vi "TLB Native Dynamic Events ver 0.05e.vi"() -> ()   [LabVIEW 2018]
uses:
  Labview Training Phase 2/Enum Controls/States for Action Engine.ctl
  Type def/TLB event states.ctl
  Type def/TLB MHL States.ctl
  <vilib>/Studica/Studica Toolkit/Background/I2C Channel.ctl
  <vilib>/Studica/Studica Toolkit/NavX/NavX.lvlib
  <vilib>/myRIO/Common/Instrument Driver Framework/myRIO v1.0/AI/typedefs/AI Channels Enum.ctl
  <vilib>/myRIO/Common/Instrument Driver Framework/myRIO v1.0/AI/typedefs/AI Channels List.ctl
  <vilib>/Studica/Studica Toolkit/Background/Mxp Selection.ctl
  <vilib>/ptbypt/NI_PtbyPt.lvlib
  Type def/Type def.ctl
  Type def/Motor Control Cluster.ctl
panel:
  out "Object detected":bool
  out "Yaw":dbl
  in  "NavX Zero Yaw":bool
  out "NavX Info Out":T2
  out "LinearAcceleration":T3
  out "Displacement":T4
  out "YRPHfH":T5
  in  "y":dbl=-1.2 format="%#_13g"
  out "Distance":T6
  in  "Return to IDLE":bool
  out "Right IR Sensor":dbl
  out "Left IR Sensor":dbl
  out "CM":fxp<+,64,16>
  out "Ultrasonic sensor":dbl format="%0.2f"
  in  "xTargetSpeed":dbl
  in  "yTargetSpeed":dbl
  in  "wTargetSpeed":dbl
  out "Speed":T7
  in  "Reset Encoder 0":bool
  out "Action Queue Items":i32
  out "State Logic Queue Items":i32
  out "Action Queues items":string[](array[string])=["Hardware reset", "Software reset", ""]
  out "State logic":T8=enum."Task 2"
  out "Action State":string
  in  "Tasks Selector":string(combo)="Task 2"
  in  "Stop Queue":bool
  in  "Start Task":bool
  # "Test Programme written by Calvin Loke    Dated: 28 Aug 2019\nTest Programme revised by Dr Alex See   Dated 30 Aug 2019\n\nProgramme version:   TLB Native Dynamic Events ver 0.04b.vi"
  # "System Health Status Update"
  # "Sequence of Actions"
  # "Continuous (Repeated)"
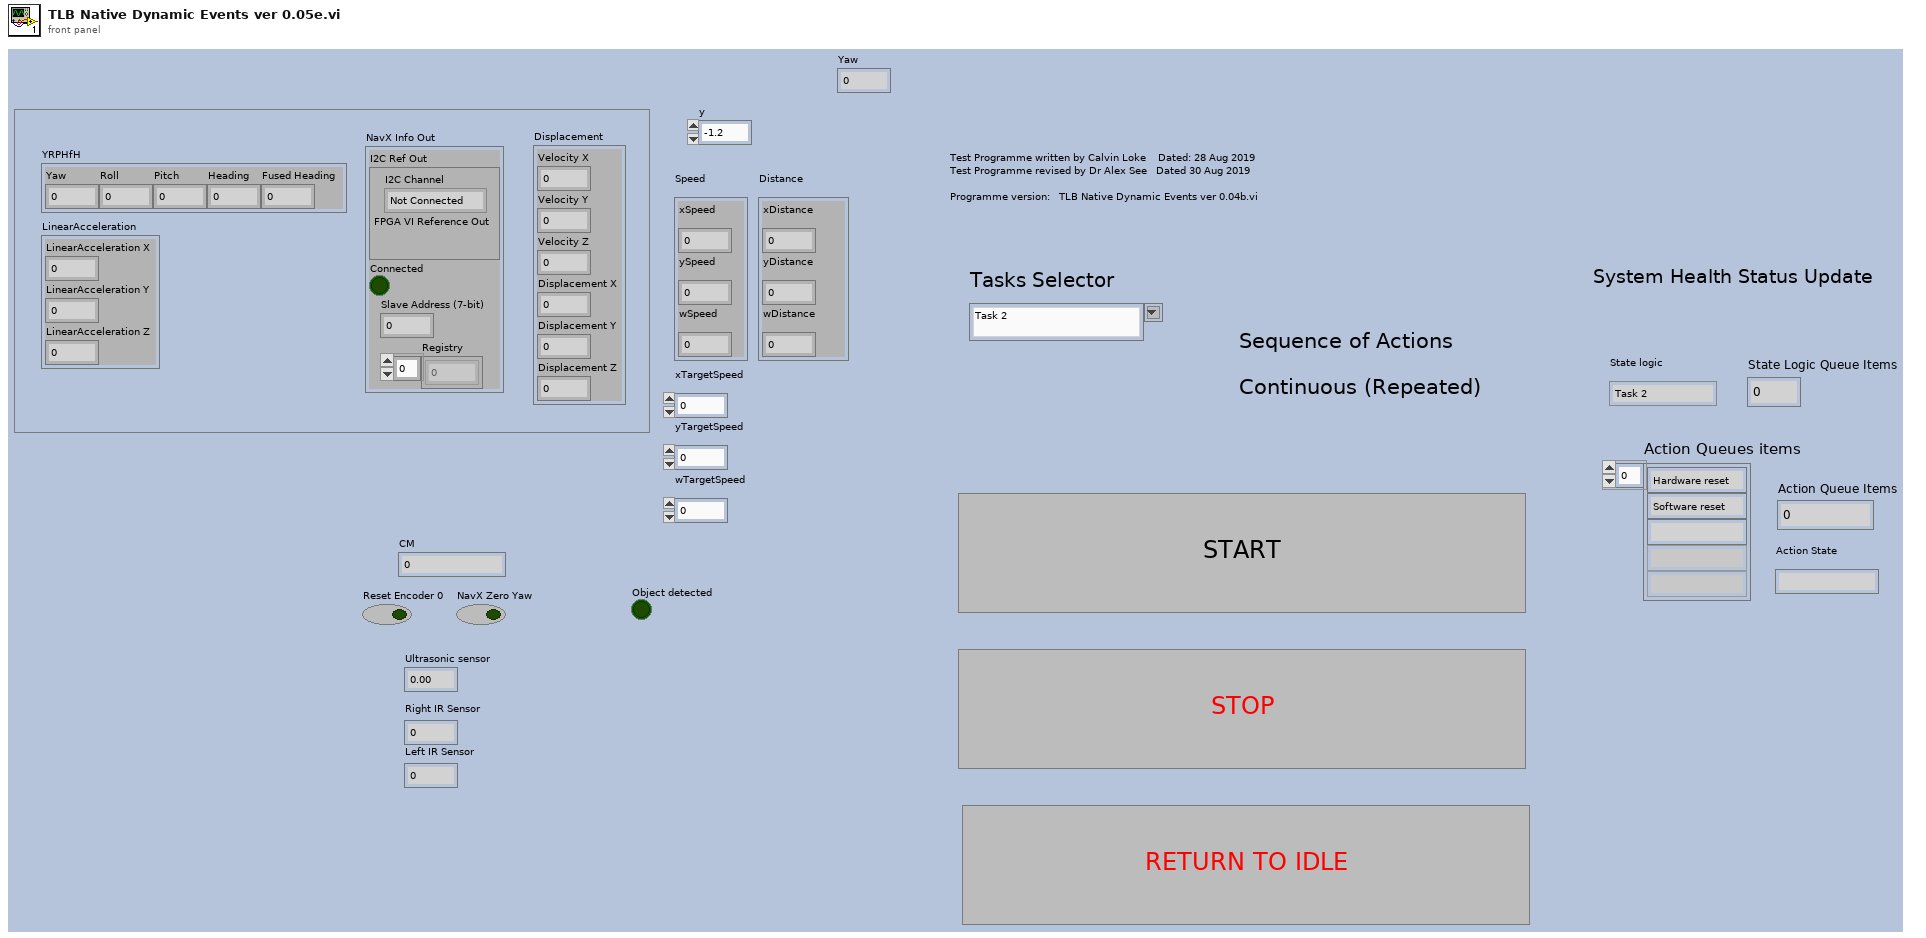
[diagram p1: front panel]
types:
  T1 = typedef "I2C Channel.ctl" = enum16{"Not Connected", "A", "B"}
  T2 = cluster{"I2C Ref Out":cluster{"I2C Channel":T1, "FPGA VI Reference Out":refnum<k20>}, "Connected":bool, "Slave Address (7-bit)":u8, "Registry":u8[]}
  T3 = cluster{"LinearAcceleration X":dbl, "LinearAcceleration Y":dbl, "LinearAcceleration Z":dbl}
  T4 = cluster{"Velocity X":dbl, "Velocity Y":dbl, "Velocity Z":dbl, "Displacement X":dbl, "Displacement Y":dbl, "Displacement Z":dbl}
  T5 = cluster{"Yaw":dbl, "Roll":dbl, "Pitch":dbl, "Heading":dbl, "Fused Heading":dbl}
  T6 = cluster{"xDistance":dbl, "yDistance":dbl, "wDistance":dbl}
  T7 = cluster{"xSpeed":dbl, "ySpeed":dbl, "wSpeed":dbl}
  T8 = typedef "TLB MHL States.ctl" = enum16{"None", "Startup", "Idle", "Processing", "Shutdown", "Reset", "Task 1", "Task 2", "Task 3", "Task 4", "Task 4a", "Task 4b", "Task 4c", "Task 4d", "Task 4e", "Task 4f", "Task 4g", "Task 4h", "Acquire image", "Wall follow mode", "Autodrive", "Autodrive a"}
  T9 = typedef "States for Action Engine.ctl" = enum16{"Initialize", "Write", "Read"}
  T10 = typedef "Motor Control Cluster.ctl" = cluster{"Vx":dbl, "Vy":dbl, "Vw":dbl}
  T11 = typedef "Type def.ctl" = cluster{"Front Ultrasonic Obstruct":bool, "Left Ultrasonic Obstruct":bool, "Right Ultrasonic Obstruct ":bool}
  T12 = typedef "TLB event states.ctl" = enum16{"Start Sequence", "Exit", "Start Task 1", "Start Task 2", "Start Task 3", "Start Task 4", "Camera vision", "Wall follow mode", "Idle", "Start Drive Straight"}
  T13 = typedef "Mxp Selection.ctl" = enum16{"MXP A", "MXP B"}
  T14 = typedef "AI Channels List.ctl" = T15[]
  T15 = typedef "AI Channels Enum.ctl" = enum16{"Not Connected", "AudioIn/Left", "AudioIn/Right", "C/AI0", "C/AI1", "A/AI0", "A/AI1", "A/AI2", "A/AI3", "A/AI4", "A/AI5", "A/AI6", "A/AI7", "B/AI0", "B/AI1", "B/AI2", "B/AI3", "B/AI4", "B/AI5", "B/AI6", "B/AI7", "AI/AI0", "AI/AI1", "AI/AI2", "AI/AI3", "A/AI0 (DIFF)", "A/AI1 (DIFF)", "A/AI2 (DIFF)", "A/AI3 (DIFF)", "B/AI0 (DIFF)", "B/AI1 (DIFF)", "B/AI2 (DIFF)", "B/AI3 (DIFF)"}
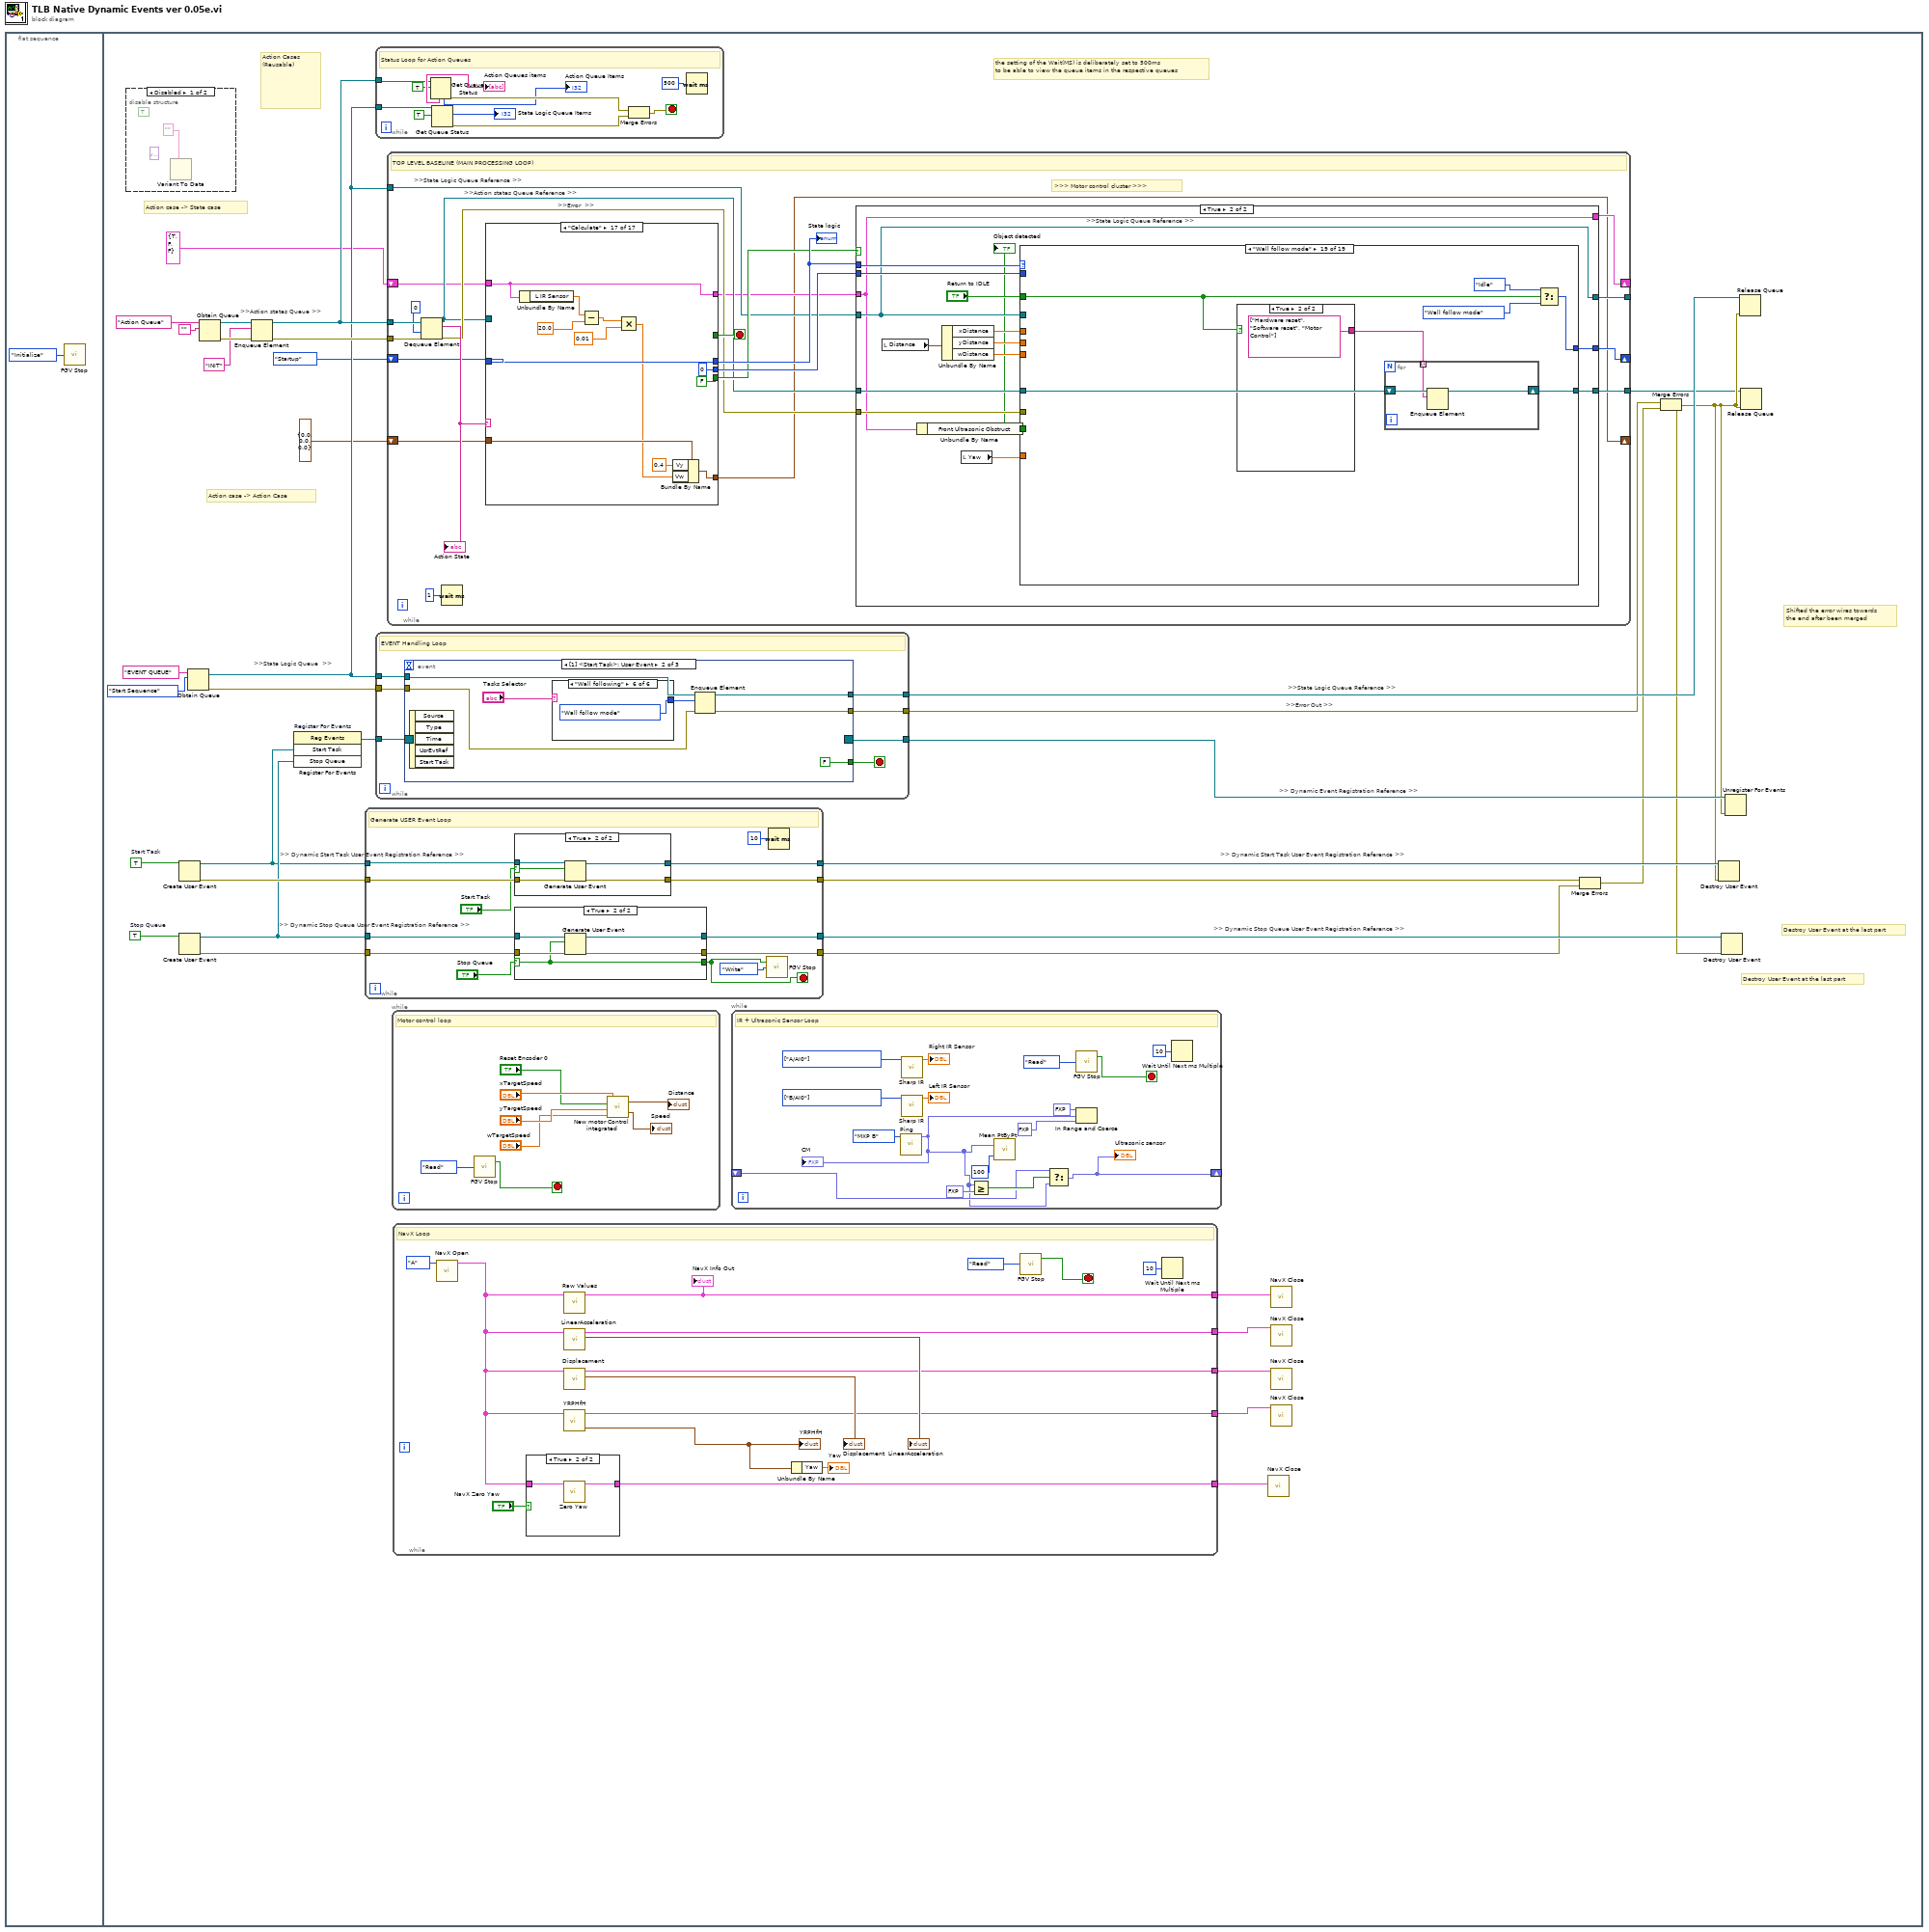
[diagram p0: block diagram]
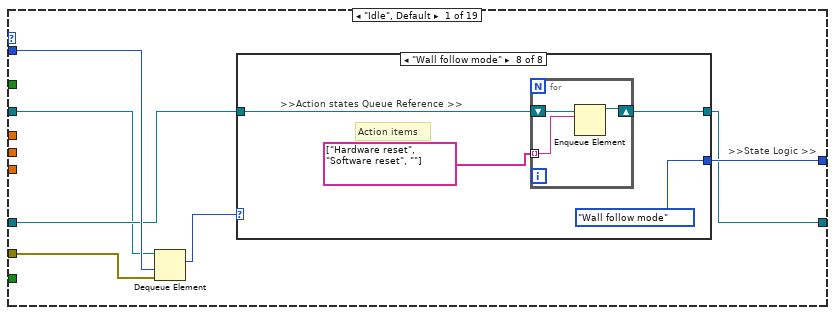
[diagram p5: hidden frame]
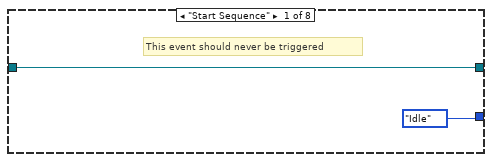
[diagram p6: hidden frame]
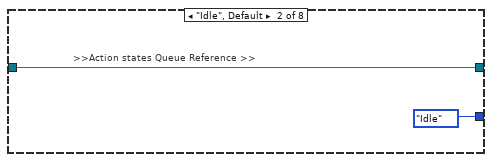
[diagram p7: hidden frame]
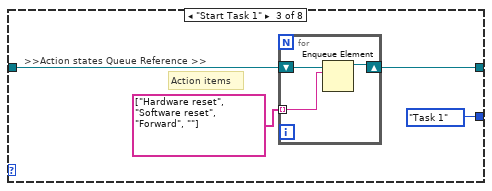
[diagram p8: hidden frame]
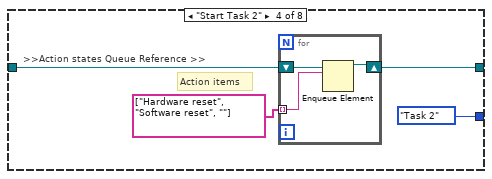
[diagram p9: hidden frame]
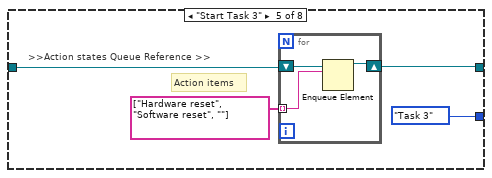
[diagram p10: hidden frame]
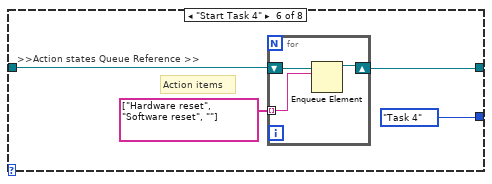
[diagram p11: hidden frame]
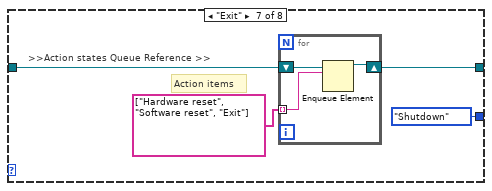
[diagram p12: hidden frame]
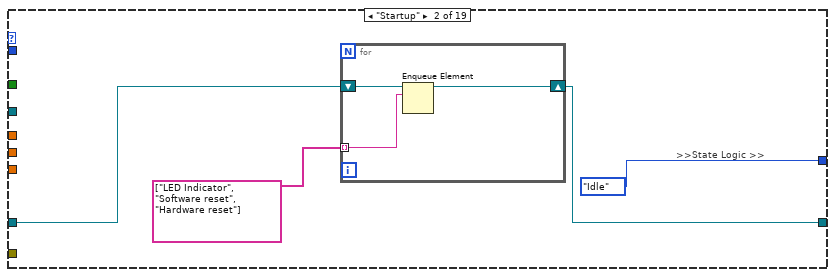
[diagram p13: hidden frame]
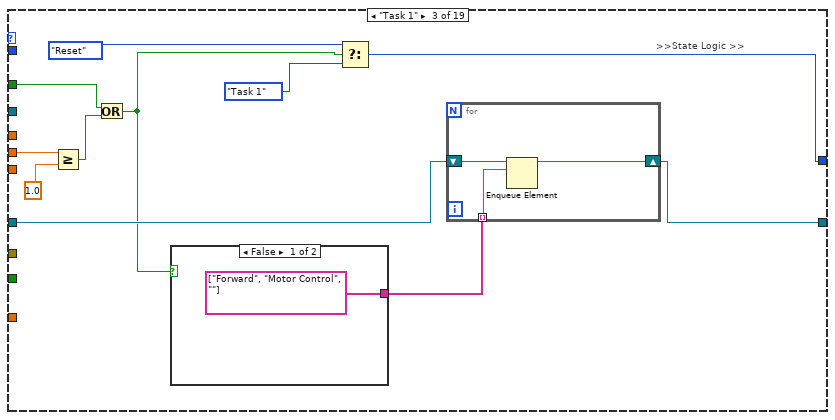
[diagram p14: hidden frame]
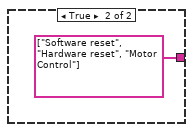
[diagram p15: hidden frame]
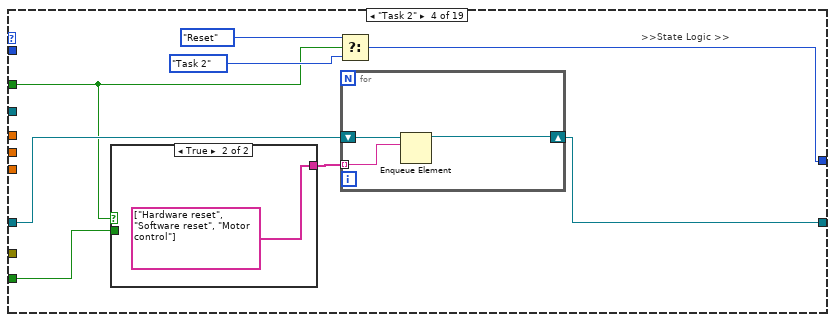
[diagram p16: hidden frame]
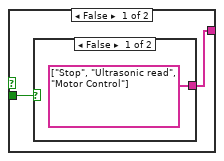
[diagram p17: hidden frame]
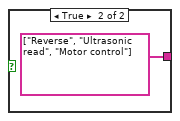
[diagram p18: hidden frame]
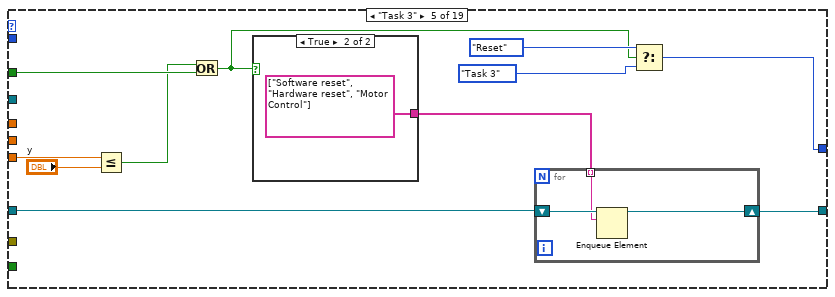
[diagram p19: hidden frame]
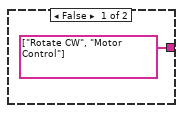
[diagram p20: hidden frame]
diagram:
  n1 = flat-sequence {
    frame #0 {
      n2 = call "FGV Stop.vi"("Init/Read/Write State"=States_for_Action_Engine."Initialize") -> ()  [unwired: 2 in, 2 out]
    }
    frame #1 {
      w37 = TRUE  # Stop Queue
      w36 = TRUE  # Start Task
      # "Action case -> Action Case"
      # "Action case -> State case"
      # "the setting of the Wait(MS) is deliberately set to 500ms\nto be able to view the queue items in the respective queues"
      # "Action Cases\n(Reusable)"
      # ">>Error Out >>"
      # ">> Dynamic Stop Queue User Event Registration Reference >>"
      # ">> Dynamic Start Task User Event Registration Reference >>"
      # ">> Dynamic Stop Queue User Event Registration Reference >>"
      # ">> Dynamic Start Task User Event Registration Reference >>"
      # ">> Dynamic Event Registration Reference >>"
      # ">>Action states Queue >>"
      # ">>State Logic Queue  >>"
      # ">>State Logic Queue Reference >>"
      # "Destroy User Event at the last part"
      # "Destroy User Event at the last part"
      # "Shifted the error wires towards\nthe end after been merged"
      n3 = disable-structure shown="Disabled" {
        frame Disabled {
          (unwired) variant
          (unwired) TRUE
          n4 = Variant To Data(type="") -> ()  [unwired: 2 in, 2 out]
        }
        frame Enabled {
        }
      }
      n5 = Create User Event(user event datatype=w36) -> (user event=w28:refnum<user-event>, error out=w33:errorcluster)  [unwired: 1 in]
      n6 = Create User Event(user event datatype=w37) -> (user event=w29:refnum<user-event>, error out=w32:errorcluster)  [unwired: 1 in]
      n7 = Obtain Queue(name (unnamed)="EVENT QUEUE", element data type=TLB_event_states."Start Sequence" ("Enum")) -> (queue out=w13:refnum<queue>, error out=w19:errorcluster)  [unwired: 3 in, 1 out]
      n8 = Obtain Queue(name (unnamed)="Action Queue", element data type="") -> (queue out=w22:refnum<queue>, error out=w18:errorcluster)  [unwired: 3 in, 1 out]
      n9 = Enqueue Element(queue=w22, element="INIT", error in (no error)=w18) -> (queue out=w14:refnum<queue>, error out=w17:errorcluster)  [unwired: 1 in, 1 out]
      n10 = register-events "Register For Events"(w28, w29) -> (reference out=w27:refnum<event-registration>)  [unwired: 2 in, 1 out]
      n11 = while {
        tunnel: w28 -> [w526]
        tunnel: w29 -> [w525]
        tunnel: [w524] -> w35
        tunnel: [w523] -> w34
        tunnel: w33 -> [w522]
        tunnel: [w521] -> w31
        tunnel: w32 -> [w520]
        tunnel: [w519] -> w30
        stop <- w515 stop-if-true
        # "Generate USER Event Loop"
        n12 = case shown="True" "Start Task" {
          selector: "Start Task" -> [_ w538]
          tunnel: w526 -> [w537 w542]
          tunnel: [w537 w541] -> w523
          tunnel: w522 -> [w536 w540]
          tunnel: [w536 w539] -> w521
          frame False {
          }
          frame True {
            n13 = Generate User Event(user event=w542, event data cluster=w538, error in=w540) -> (user event out=w541:refnum<user-event>, error out=w539:errorcluster)  [unwired: 1 in]
          }
        }
        n14 = case shown="True" "Stop Queue" {
          selector: "Stop Queue" -> [_ w531]
          tunnel: w525 -> [w530 w535]
          tunnel: [w530 w534] -> w524
          tunnel: w520 -> [w529 w533]
          tunnel: [w529 w532] -> w519
          tunnel: [FALSE w531] -> w515
          frame False {
          }
          frame True {
            n15 = Generate User Event(user event=w535, event data cluster=w531, error in=w533) -> (user event out=w534:refnum<user-event>, error out=w532:errorcluster)  [unwired: 1 in]
          }
        }
        n16 = call "FGV Stop.vi"("Init/Read/Write State"=States_for_Action_Engine."Write", "Input Node"=w515) -> ()  [unwired: 1 in, 2 out]
        n17 = Wait (ms)(milliseconds to wait=u32 10) -> ()  [unwired: 1 out]
      }
      n18 = while {
        tunnel: w14 -> [w89]
        tunnel: w13 -> [w86]
        stop <- w83 stop-if-true
        # "Status Loop for Action Queues"
        n19 = Get Queue Status(queue=w89, return elements? (F)=TRUE) -> (error out=w85:errorcluster, # elements in queue=→"Action Queue Items":i32, elements=→"Action Queues items":string[])  [unwired: 1 in, 5 out]
        n20 = Get Queue Status(queue=w86, return elements? (F)=TRUE) -> (# pending remove=→"State Logic Queue Items":i32, error out=w84:errorcluster)  [unwired: 1 in, 6 out]
        n21 = Merge Errors(w85, w84) -> (w83:errorcluster)
        n22 = Wait (ms)(milliseconds to wait=u32 500) -> ()  [unwired: 1 out]
      }
      n23 = while {
        tunnel: w27 -> [w489]
        tunnel: [w488] -> w26
        tunnel: w13 -> [w486]
        tunnel: [w485] -> w25
        tunnel: w19 -> [w484]
        tunnel: [w483] -> w16
        stop <- w487 stop-if-true
        # "EVENT Handling Loop"
        n24 = event shown="[1] <Start Task>: User Event" {
          selector: w489 -> [_ _ _]
          dyn-events: [_ _ _] -> w488
          timeout: _ -> [_ _ _]
          tunnel: [FALSE FALSE w514] -> w487
          tunnel: w486 -> [w494 w501 w512]
          tunnel: [w493 w500 w513] -> w485
          tunnel: w484 -> [w491 w497 w510]
          tunnel: [w490 w496 w509] -> w483
          event Timeout {
            n25 = event-data() -> ()  [unwired: 1 in, 3 out]
            n26 = Enqueue Element(queue=w494, element=TLB_event_states."Idle" ("Enum"), error in (no error)=w491) -> (queue out=w493:refnum<queue>, error out=w490:errorcluster)  [unwired: 1 in, 1 out]
          }
          event User Event {
            n27 = event-data() -> ()  [unwired: 1 in, 5 out]
            n28 = case shown="\"Wall following\"" "Tasks Selector" {
              tunnel: [TLB_event_states."Idle" ("Enum") TLB_event_states."Start Task 1" ("Enum") TLB_event_states."Start Task 2" ("Enum") TLB_event_states."Start Task 3" ("Enum") TLB_event_states."Start Task 4" ("Enum") TLB_event_states."Wall follow mode" ("Enum")] -> w498
              frame Default {
              }
              frame "Task 1" {
              }
              frame "Task 2" {
              }
              frame "Task 3" {
              }
              frame "Task 4" {
              }
              frame "Wall following" {
              }
            }
            n29 = Enqueue Element(queue=w501, element=w498, error in (no error)=w497) -> (queue out=w500:refnum<queue>, error out=w496:errorcluster)  [unwired: 1 in, 1 out]
          }
          event User Event {
            n30 = event-data() -> ("Stop Queue"=w514:bool)  [unwired: 1 in, 4 out]
            n31 = Enqueue Element At Opposite End(queue=w512, element=TLB_event_states."Exit" ("Enum"), error in (no error)=w510) -> (queue out=w513:refnum<queue>, error out=w509:errorcluster)  [unwired: 1 in, 1 out]
          }
        }
      }
      n32 = while {
        tunnel: w13 -> [w100]
        shift-right: [w105] -> _
        shift-left: TLB_MHL_States."Startup" ("Enum") -> [w97]
        tunnel: w14 -> [w110]
        tunnel: w17 -> [w108]
        tunnel: [w107] -> _
        tunnel: [w106] -> w11
        shift-right: [w94] -> _
        shift-left: T11 {"Front Ultrasonic Obstruct"=TRUE, "Left Ultrasonic Obstruct"=FALSE, "Right Ultrasonic Obstruct "=FALSE} -> [w96]
        shift-right: [w92] -> _
        shift-left: T10 {"Vx"=0.0, "Vy"=0.0, "Vw"=0.0} -> [w93]
        stop <- w103 stop-if-true
        # ">>> Motor control cluster >>>"
        # ">>Error  >>"
        # ">>Action states Queue Reference >>"
        # ">>State Logic Queue Reference >>"
        # "TOP LEVEL BASELINE (MAIN PROCESSING LOOP)"
        n33 = Dequeue Element(queue=w110, timeout in ms (-1)=0, error in (no error)=w108) -> (queue out=w98:refnum<queue>, element=w109:string, error out=w99:errorcluster)  [unwired: 1 out]
        "Action State" <- w109
        n34 = Wait (ms)(milliseconds to wait=u32 1) -> ()  [unwired: 1 out]
        n35 = case shown="\"Calculate\"" w109 {
          tunnel: [w349 w356 w361 w369 w378 w388 w397 w404 w415 w423 w431 w439 w448 TLB_MHL_States."Shutdown" ("Enum") w463 w467 w481] -> w111
          tunnel: [w348 0 0 0 0 0 0 0 0 0 0 0 0 0 0 0 0] -> w104
          tunnel: [_ _ _ _ _ _ _ _ _ _ _ _ _ TRUE _ _ _] -> w103
          tunnel: [TRUE FALSE FALSE FALSE FALSE FALSE FALSE FALSE FALSE FALSE FALSE FALSE FALSE FALSE FALSE FALSE FALSE] -> w102
          tunnel: w98 -> [_ _ _ _ _ _ _ _ _ _ _ _ _ _ _ _ _]
          tunnel: w97 -> [w349 w356 w361 w369 w378 w388 w397 w404 w415 w423 w431 w439 w448 _ w463 w467 w481]
          tunnel: w96 -> [w346 w353 w358 w365 w374 w383 w392 w401 w410 w419 w432 w436 w443 w450 w462 w470 w482]
          tunnel: [w346 w353 w358 w365 w374 w383 w392 w401 w410 w419 w432 w435 w443 w450 w459 w469 w482] -> w95
          tunnel: w93 -> [w345 w352 w357 w363 w372 w381 w391 w399 w409 w417 w425 w433 w442 w449 w455 w464 w473]
          tunnel: [w345 w352 w357 w364 w373 w382 w390 w400 w408 w418 w425 w433 w440 w449 w455 w464 w474] -> w92
          frame "No action", Default {
            n36 = case shown="\"Idle\"" w349 {
              tunnel: [0 100] -> w348
              frame "Startup", Default {
              }
              frame "Idle" {
              }
            }
          }
          frame "Init" {
            # ">>State Logic  >>"
          }
          frame "LED Indicator" {
          }
          frame "Forward" {
            n37 = local write "Reset Encoder 0"(FALSE ("Reset Encoder 0")) -> ()
            n38 = local write "NavX Zero Yaw"(FALSE ("NavX Zero Yaw")) -> ()
            n39 = Bundle By Name(cluster=w363, "Vy"=0.6) -> (w364:T10)
          }
          frame "Reverse" {
            n40 = local write "NavX Zero Yaw"(FALSE ("NavX Zero Yaw")) -> ()
            n41 = local write "Reset Encoder 0"(FALSE ("Reset Encoder 0")) -> ()
            n42 = Bundle By Name(cluster=w372, "Vy"=-0.6) -> (w373:T10)
          }
          frame "Right" {
            n43 = local write "NavX Zero Yaw"(FALSE ("NavX Zero Yaw")) -> ()
            n44 = local write "Reset Encoder 0"(FALSE ("Reset Encoder 0")) -> ()
            n45 = Bundle By Name(cluster=w381, "Vx"=0.6) -> (w382:T10)
          }
          frame "Left" {
            n46 = Bundle By Name(cluster=w391, "Vx"=-0.6) -> (w390:T10)
            n47 = local write "NavX Zero Yaw"(FALSE ("NavX Zero Yaw")) -> ()
            n48 = local write "Reset Encoder 0"(FALSE ("Reset Encoder 0")) -> ()
          }
          frame "Rotate CW" {
            n49 = local write "NavX Zero Yaw"(FALSE ("NavX Zero Yaw")) -> ()
            n50 = local write "Reset Encoder 0"(FALSE ("Reset Encoder 0")) -> ()
            n51 = Bundle By Name(cluster=w399, "Vw"=-0.3) -> (w400:T10)
          }
          frame "Rotate ACW" {
            n52 = local write "Reset Encoder 0"(FALSE ("Reset Encoder 0")) -> ()
            n53 = local write "NavX Zero Yaw"(FALSE ("NavX Zero Yaw")) -> ()
            n54 = Bundle By Name(cluster=w409, "Vw"=0.15) -> (w408:T10)
          }
          frame "Stop" {
            w416 = 0.0
            n55 = local write "NavX Zero Yaw"(FALSE ("NavX Zero Yaw")) -> ()
            n56 = local write "Reset Encoder 0"(FALSE ("Reset Encoder 0")) -> ()
            n57 = Bundle By Name(cluster=w417, "Vx"=w416, "Vy"=w416, "Vw"=w416) -> (w418:T10)
          }
          frame "Motor control" {
            # "Replace with FGV"
            n58 = Unbundle By Name(w425) -> ("Vx"=w428:dbl, "Vy"=w427:dbl, "Vw"=w426:dbl)
            n59 = local write "xTargetSpeed"(w428) -> ()
            n60 = local write "yTargetSpeed"(w427) -> ()
            n61 = local write "wTargetSpeed"(w426) -> ()
          }
          frame "Software reset" {
            w434 = FALSE ("NavX Zero Yaw")
            n62 = local write "NavX Zero Yaw"(w434) -> ()
            n63 = Bundle By Name(cluster=w436, "Front Ultrasonic Obstruct"=w434) -> (w435:T11)
          }
          frame "Hardware reset" {
            w441 = 0.0
            n64 = local write "Reset Encoder 0"(TRUE ("Reset Encoder 0")) -> ()
            n65 = local write "NavX Zero Yaw"(TRUE ("NavX Zero Yaw")) -> ()
            n66 = Bundle By Name(cluster=w442, "Vx"=w441, "Vy"=w441, "Vw"=w441) -> (w440:T10)
          }
          frame "Exit" {
          }
          frame "Ultrasonic read" {
            # "Object detection"
            n67 = local read "Ultrasonic sensor"() -> (w458:dbl)
            n68 = Less Or Equal?(x=w458, y=20.0) -> (x <= y?=w456:bool)
            n69 = Bundle By Name(cluster=w462, "Front Ultrasonic Obstruct"=w456) -> (w459:T11)
          }
          frame "IR Sensor Read" {
            n70 = local read "Left IR Sensor"() -> (w468:dbl)
            n71 = Bundle By Name(cluster=w470, "L IR Sensor"=w468) -> (w469:T11)
          }
          frame "Calculate" {
            n72 = Unbundle By Name(w482) -> ("L IR Sensor"=w478:dbl)
            n73 = Subtract(x=w478, y=20.0) -> (x-y=w476:dbl)
            n74 = Multiply(x=w476, y=0.01) -> (x*y=w472:dbl)
            n75 = Bundle By Name(cluster=w473, "Vy"=0.4, "Vw"=w472) -> (w474:T10)
          }
        }
        "State logic" <- w111
        n76 = case shown="True" w102 {
          tunnel: w111 -> [w115 w131]
          tunnel: w100 -> [w116 w125]
          tunnel: w98 -> [w114 w130]
          tunnel: [w116 w125] -> w107
          tunnel: [w114 w129] -> w106
          tunnel: [w115 w128] -> w105
          tunnel: w99 -> [_ w127]
          tunnel: w104 -> [_ w126]
          tunnel: w95 -> [w113 w117]
          tunnel: [w113 w117] -> w94
          frame False {
          }
          frame True {
            # ">>State Logic Queue Reference >>"
            n77 = local read "Distance"() -> (w123:T6)
            n78 = Unbundle By Name(w117) -> ("Front Ultrasonic Obstruct"=w118:bool)
            "Object detected" <- w118
            n79 = Unbundle By Name(w123) -> ("xDistance"=w120:dbl, "yDistance"=w122:dbl, "wDistance"=w121:dbl)
            n80 = local read "Yaw"() -> (w119:dbl)
            n81 = case shown="\"Wall follow mode\"" w131 {
              tunnel: w125 -> [w132 _ _ _ _ _ _ _ _ _ _ _ _ _ _ _ _ _ _]
              tunnel: w130 -> [w134 w186 w198 w211 w233 w242 w256 w271 w284 w297 w308 w314 w317 w323 w326 w328 w330 w332 w335]
              tunnel: [w133 w185 w197 w212 w232 w243 w255 w270 w283 w296 w307 w314 w316 w323 w326 w328 w330 w332 w336] -> w129
              tunnel: [w137 TLB_MHL_States."Idle" ("Enum") w200 w213 w229 w246 w258 w269 w285 w295 TLB_MHL_States."Idle" ("Enum") TLB_MHL_States."Reset" ("Enum") TLB_MHL_States."Shutdown" ("Enum") TLB_MHL_States."Reset" ("Enum") TLB_MHL_States."Idle" ("Enum") TLB_MHL_States."Idle" ("Enum") TLB_MHL_States."Idle" ("Enum") TLB_MHL_States."Idle" ("Enum") w338] -> w128
              tunnel: w127 -> [w135 _ _ _ _ _ _ _ _ _ _ _ _ _ _ _ _ _ _]
              tunnel: w126 -> [w136 _ _ _ _ _ _ _ _ _ _ _ _ _ _ _ _ _ _]
              tunnel: "Return to IDLE" -> [_ _ w195 w210 w227 _ _ _ _ _ _ _ _ _ _ _ _ _ w333]
              tunnel: w122 -> [_ _ w194 _ _ _ _ w268 _ _ _ _ _ _ _ _ _ _ _]
              tunnel: w121 -> [_ _ _ _ w226 _ _ _ _ _ _ _ _ _ _ _ _ _ _]
              tunnel: w120 -> [_ _ _ _ _ _ w252 _ w280 _ _ _ _ _ _ _ _ _ _]
              tunnel: w119 -> [_ _ _ _ _ _ _ _ _ _ _ _ _ _ _ _ _ _ _]
              tunnel: w118 -> [_ _ _ w208 _ w240 _ _ _ w294 _ _ _ _ _ _ _ _ _]
              frame "Idle", Default {
                # ">>State Logic >>"
                n82 = Dequeue Element(queue=w132, timeout in ms (-1)=w136, error in (no error)=w135) -> (element=w138:T12)  [unwired: 3 out]
                n83 = case shown="\"Wall follow mode\"" w138 {
                  tunnel: [TLB_MHL_States."Idle" ("Enum") TLB_MHL_States."Idle" ("Enum") TLB_MHL_States."Task 1" ("Enum") TLB_MHL_States."Task 2" ("Enum") TLB_MHL_States."Task 3" ("Enum") TLB_MHL_States."Task 4" ("Enum") TLB_MHL_States."Shutdown" ("Enum") TLB_MHL_States."Wall follow mode" ("Enum")] -> w137
                  tunnel: [w140 w141 w145 w150 w159 w165 w171 w178] -> w133
                  tunnel: w134 -> [w140 w141 w143 w151 w160 w166 w172 w179]
                  frame "Start Sequence" {
                    # "This event should never be triggered"
                  }
                  frame "Idle", Default {
                    # ">>Action states Queue Reference >>"
                  }
                  frame "Start Task 1" {
                    # ">>Action states Queue Reference >>"
                    # "Action items"
                    n84 = for {
                      shift-right: [w149] -> w145
                      shift-left: w143 -> [w148]
                      tunnel: string[] ["Hardware reset", "Software reset", "Forward", ""] -> [w147] mode=indexing
                      n85 = Enqueue Element(queue=w148, element=w147) -> (queue out=w149:refnum<queue>)  [unwired: 2 in, 2 out]
                    }
                  }
                  frame "Start Task 2" {
                    # ">>Action states Queue Reference >>"
                    # "Action items"
                    n86 = for {
                      shift-right: [w156] -> w150
                      shift-left: w151 -> [w155]
                      tunnel: string[] ["Hardware reset", "Software reset", ""] -> [w154] mode=indexing
                      n87 = Enqueue Element(queue=w155, element=w154) -> (queue out=w156:refnum<queue>)  [unwired: 2 in, 2 out]
                    }
                  }
                  frame "Start Task 3" {
                    # ">>Action states Queue Reference >>"
                    # "Action items"
                    n88 = for {
                      shift-right: [w163] -> w159
                      shift-left: w160 -> [w162]
                      tunnel: string[] ["Hardware reset", "Software reset", ""] -> [w161] mode=indexing
                      n89 = Enqueue Element(queue=w162, element=w161) -> (queue out=w163:refnum<queue>)  [unwired: 2 in, 2 out]
                    }
                  }
                  frame "Start Task 4" {
                    # ">>Action states Queue Reference >>"
                    # "Action items"
                    n90 = for {
                      shift-right: [w170] -> w165
                      shift-left: w166 -> [w169]
                      tunnel: string[] ["Hardware reset", "Software reset", ""] -> [w168] mode=indexing
                      n91 = Enqueue Element(queue=w169, element=w168) -> (queue out=w170:refnum<queue>)  [unwired: 2 in, 2 out]
                    }
                  }
                  frame "Exit" {
                    # ">>Action states Queue Reference >>"
                    # "Action items"
                    n92 = for {
                      shift-right: [w177] -> w171
                      shift-left: w172 -> [w176]
                      tunnel: string[] ["Hardware reset", "Software reset", "Exit"] -> [w175] mode=indexing
                      n93 = Enqueue Element(queue=w176, element=w175) -> (queue out=w177:refnum<queue>)  [unwired: 2 in, 2 out]
                    }
                  }
                  frame "Wall follow mode" {
                    # ">>Action states Queue Reference >>"
                    # "Action items"
                    n94 = for {
                      shift-right: [w184] -> w178
                      shift-left: w179 -> [w183]
                      tunnel: string[] ["Hardware reset", "Software reset", ""] -> [w182] mode=indexing
                      n95 = Enqueue Element(queue=w183, element=w182) -> (queue out=w184:refnum<queue>)  [unwired: 2 in, 2 out]
                    }
                  }
                }
              }
              frame "Startup" {
                # ">>State Logic >>"
                n96 = for {
                  shift-right: [w190] -> w185
                  shift-left: w186 -> [w191]
                  tunnel: string[] ["LED Indicator", "Software reset", "Hardware reset"] -> [w189] mode=indexing
                  n97 = Enqueue Element(queue=w191, element=w189) -> (queue out=w190:refnum<queue>)  [unwired: 2 in, 2 out]
                }
              }
              frame "Task 1" {
                # ">>State Logic >>"
                n98 = Greater Or Equal?(x=w194, y=1.0) -> (x >= y?=w192:bool)
                n99 = Or(x=w195, y=w192) -> (x .or. y?=w196:bool)
                n100 = case shown="False" w196 {
                  tunnel: [string[] ["Forward", "Motor Control", ""] string[] ["Software reset", "Hardware reset", "Motor Control"]] -> w199
                  frame False {
                  }
                  frame True {
                  }
                }
                n101 = Select(t=TLB_MHL_States."Reset" ("Enum"), s=w196, f=TLB_MHL_States."Task 1" ("Enum")) -> (s? t:f=w200:T8)
                n102 = for {
                  shift-right: [w206] -> w197
                  shift-left: w198 -> [w207]
                  tunnel: w199 -> [w205] mode=indexing
                  n103 = Enqueue Element(queue=w207, element=w205) -> (queue out=w206:refnum<queue>)  [unwired: 2 in, 2 out]
                }
              }
              frame "Task 2" {
                # ">>State Logic >>"
                n104 = case shown="True" w210 {
                  tunnel: [w217 string[] ["Hardware reset", "Software reset", "Motor control"]] -> w209
                  tunnel: w208 -> [w216 _]
                  frame False {
                    n105 = case shown="False" w216 {
                      tunnel: [string[] ["Stop", "Ultrasonic read", "Motor Control"] string[] ["Reverse", "Ultrasonic read", "Motor control"]] -> w217
                      frame False {
                      }
                      frame True {
                      }
                    }
                  }
                  frame True {
                  }
                }
                n106 = Select(t=TLB_MHL_States."Reset" ("Enum"), s=w210, f=TLB_MHL_States."Task 2" ("Enum")) -> (s? t:f=w213:T8)
                n107 = for {
                  shift-right: [w222] -> w212
                  shift-left: w211 -> [w223]
                  tunnel: w209 -> [w221] mode=indexing
                  n108 = Enqueue Element(queue=w223, element=w221) -> (queue out=w222:refnum<queue>)  [unwired: 2 in, 2 out]
                }
              }
              frame "Task 3" {
                n109 = Less Or Equal?(x=w226, y="y") -> (x <= y?=w224:bool)
                n110 = Or(x=w224, y=w227) -> (x .or. y?=w228:bool)
                n111 = case shown="True" w228 {
                  tunnel: [string[] ["Rotate CW", "Motor Control"] string[] ["Software reset", "Hardware reset", "Motor Control"]] -> w234
                  frame False {
                  }
                  frame True {
                  }
                }
                n112 = for {
                  shift-right: [w236] -> w232
                  shift-left: w233 -> [w237]
                  tunnel: w234 -> [w235] mode=indexing
                  n113 = Enqueue Element(queue=w237, element=w235) -> (queue out=w236:refnum<queue>)  [unwired: 2 in, 2 out]
                }
                n114 = Select(t=TLB_MHL_States."Reset" ("Enum"), s=w228, f=TLB_MHL_States."Task 3" ("Enum")) -> (s? t:f=w229:T8)
              }
              frame "Task 4" {
                n115 = case shown="False" w240 {
                  tunnel: [string[] ["Forward", "Ultrasonic read", "Motor Control"] string[] ["Stop", "Hardware reset", "Software reset", "Motor Control"]] -> w241
                  frame False {
                  }
                  frame True {
                  }
                }
                n116 = for {
                  shift-right: [w250] -> w243
                  shift-left: w242 -> [w251]
                  tunnel: w241 -> [w249] mode=indexing
                  n117 = Enqueue Element(queue=w251, element=w249) -> (queue out=w250:refnum<queue>)  [unwired: 2 in, 2 out]
                }
                n118 = Select(t=TLB_MHL_States."Task 4a" ("Enum"), s=w240, f=TLB_MHL_States."Task 4" ("Enum")) -> (s? t:f=w246:T8)
              }
              frame "Task 4a" {
                n119 = Greater Or Equal?(x=w252, y=0.5) -> (x >= y?=w254:bool)
                n120 = case shown="True" w254 {
                  tunnel: [string[] ["Right", "Motor Control"] string[] ["Stop", "Hardware reset", "Software reset", "Motor Control"]] -> w257
                  frame False {
                  }
                  frame True {
                  }
                }
                n121 = for {
                  shift-right: [w264] -> w255
                  shift-left: w256 -> [w265]
                  tunnel: w257 -> [w263] mode=indexing
                  n122 = Enqueue Element(queue=w265, element=w263) -> (queue out=w264:refnum<queue>)  [unwired: 2 in, 2 out]
                }
                n123 = Select(t=TLB_MHL_States."Task 4b" ("Enum"), s=w254, f=TLB_MHL_States."Task 4a" ("Enum")) -> (s? t:f=w258:T8)
              }
              frame "Task 4b" {
                n124 = Greater Or Equal?(x=w268, y=0.75) -> (x >= y?=w266:bool)
                n125 = case shown="False" w266 {
                  tunnel: [string[] ["Forward"] string[] ["Stop", "Hardware reset", "Software reset"]] -> w272
                  frame False {
                  }
                  frame True {
                  }
                }
                n126 = for {
                  shift-right: [w278] -> w270
                  shift-left: w271 -> [w279]
                  tunnel: w272 -> [w277] mode=indexing
                  n127 = Enqueue Element(queue=w279, element=w277) -> (queue out=w278:refnum<queue>)  [unwired: 2 in, 2 out]
                }
                n128 = Select(t=TLB_MHL_States."Task 4c" ("Enum"), s=w266, f=TLB_MHL_States."Task 4b" ("Enum")) -> (s? t:f=w269:T8)
              }
              frame "Task 4c" {
                n129 = Less Or Equal?(x=w280, y=-0.65) -> (x <= y?=w281:bool)
                n130 = case shown="False" w281 {
                  tunnel: [string[] ["Left"] string[] ["Stop", "Hardware reset", "Software reset"]] -> w286
                  frame False {
                  }
                  frame True {
                  }
                }
                n131 = for {
                  shift-right: [w292] -> w283
                  shift-left: w284 -> [w293]
                  tunnel: w286 -> [w291] mode=indexing
                  n132 = Enqueue Element(queue=w293, element=w291) -> (queue out=w292:refnum<queue>)  [unwired: 2 in, 2 out]
                }
                n133 = Select(t=TLB_MHL_States."Task 4d" ("Enum"), s=w281, f=TLB_MHL_States."Task 4c" ("Enum")) -> (s? t:f=w285:T8)
              }
              frame "Task 4d" {
                n134 = case shown="False" w294 {
                  tunnel: [string[] ["Forward", "Ultrasonic Read"] string[] ["Stop", "Hardware reset", "Software reset"]] -> w298
                  frame False {
                  }
                  frame True {
                  }
                }
                n135 = for {
                  shift-right: [w304] -> w296
                  shift-left: w297 -> [w305]
                  tunnel: w298 -> [w303] mode=indexing
                  n136 = Enqueue Element(queue=w305, element=w303) -> (queue out=w304:refnum<queue>)  [unwired: 2 in, 2 out]
                }
                n137 = Select(t=TLB_MHL_States."Task 4e" ("Enum"), s=w294, f=TLB_MHL_States."Task 4d" ("Enum")) -> (s? t:f=w295:T8)
              }
              frame "Reset" {
                n138 = for {
                  shift-right: [w312] -> w307
                  shift-left: w308 -> [w313]
                  tunnel: string[] ["Software reset", "Hardware reset", ""] -> [w311] mode=indexing
                  n139 = Enqueue Element(queue=w313, element=w311) -> (queue out=w312:refnum<queue>)  [unwired: 2 in, 2 out]
                }
                n140 = Wait (ms)(milliseconds to wait=u32 250) -> ()  [unwired: 1 out]
              }
              frame "Processing" {
              }
              frame "Shutdown" {
                # ">>State Logic >>"
                n141 = for {
                  shift-right: [w321] -> w316
                  shift-left: w317 -> [w322]
                  tunnel: string[] ["Software reset", "Hardware reset", "Exit"] -> [w320] mode=indexing
                  n142 = Enqueue Element(queue=w322, element=w320) -> (queue out=w321:refnum<queue>)  [unwired: 2 in, 2 out]
                }
              }
              frame "None" {
              }
              frame "Task 4e" {
              }
              frame "Task 4f" {
              }
              frame "Task 4g" {
              }
              frame "Task 4h" {
              }
              frame "Wall follow mode" {
                n143 = case shown="True" w333 {
                  tunnel: [string[] ["IR Sensor Read", "Calculate", "Forward", "Motor Control"] string[] ["Hardware reset", "Software reset", "Motor Control"]] -> w334
                  frame False {
                  }
                  frame True {
                  }
                }
                n144 = for {
                  shift-right: [w343] -> w336
                  shift-left: w335 -> [w344]
                  tunnel: w334 -> [w342] mode=indexing
                  n145 = Enqueue Element(queue=w344, element=w342) -> (queue out=w343:refnum<queue>)  [unwired: 2 in, 2 out]
                }
                n146 = Select(t=TLB_MHL_States."Idle" ("Enum"), s=w333, f=TLB_MHL_States."Wall follow mode" ("Enum")) -> (s? t:f=w338:T8)
              }
            }
          }
        }
      }
      n147 = while {
        stop <- w79 stop-if-true
        # "Motor control loop"
        n148 = call "FGV Stop.vi"("Init/Read/Write State"=States_for_Action_Engine."Read") -> ("Output node"=w79:bool)  [unwired: 2 in, 1 out]
        n149 = call "New motor Control integrated.vi"("wTargetSpeed"="wTargetSpeed", "yTargetSpeed"="yTargetSpeed", "xTargetSpeed"="Reset Encoder 0", "Reset Encoders"="xTargetSpeed") -> ("Speed"=→"Speed":T7, "Distance"=→"Distance":T6)
      }
      n150 = while {
        tunnel: [w49] -> w7
        tunnel: [w46] -> w6
        tunnel: [w45] -> w4
        tunnel: [w44] -> w5
        tunnel: [w41] -> w3
        stop <- w51 stop-if-true
        # "NavX Loop"
        n151 = call <vilib>:"NavX Open.vi"("I2C Channel"=I2C_Channel."A") -> ("NavX Info"=w42:T2)  [unwired: 9 in, 1 out]
        n152 = case shown="True" "NavX Zero Yaw" {
          tunnel: w42 -> [w53 w55]
          tunnel: [w53 w54] -> w41
          frame False {
          }
          frame True {
            n153 = call <vilib>:"Zero Yaw.vi"("NavX Info In"=w55) -> ("NavX Info Out"=w54:T2)  [unwired: 10 in]
          }
        }
        n154 = call <vilib>:"YRPHfH.vi"("NavX Info In"=w42) -> ("YRPHfH"=w39:T5, "NavX Info Out"=w45:T2)  [unwired: 3 in]
        "YRPHfH" <- w39
        n155 = call <vilib>:"Raw Values.vi"("NavX Info In"=w42) -> ("NavX Info Out"=w49:T2)  [unwired: 8 in, 1 out]
        "NavX Info Out" <- w49
        n156 = call <vilib>:"LinearAcceleration.vi"("NavX Info In"=w42) -> ("LinearAcceleration"=→"LinearAcceleration":T3, "NavX Info Out"=w46:T2)  [unwired: 9 in]
        n157 = call <vilib>:"Displacement.vi"("NavX Info In"=w42) -> ("Displacement"=→"Displacement":T4, "NavX Info Out"=w44:T2)  [unwired: 9 in]
        n158 = Unbundle By Name(w39) -> ("Yaw"=→"Yaw":dbl)
        n159 = call "FGV Stop.vi"("Init/Read/Write State"=States_for_Action_Engine."Read") -> ("Output node"=w51:bool)  [unwired: 2 in, 1 out]
        n160 = Wait Until Next ms Multiple(millisecond multiple=u32 10) -> ()  [unwired: 1 out]
      }
      n161 = while {
        shift-right: [w60] -> _
        shift-left: _ -> [w61]
        stop <- w66 stop-if-true
        w71 = T14 [enum."B/AI0"] items=["Not Connected", "AudioIn/Left", "AudioIn/Right", "C/AI0", "C/AI1", "A/AI0", "A/AI1", "A/AI2", "A/AI3", "A/AI4", "A/AI5", "A/AI6", "A/AI7", "B/AI0", "B/AI1", "B/AI2", "B/AI3", "B/AI4", "B/AI5", "B/AI6", "B/AI7", "AI/AI0", "AI/AI1", "AI/AI2", "AI/AI3", "A/AI0 (DIFF)", "A/AI1 (DIFF)", "A/AI2 (DIFF)", "A/AI3 (DIFF)", "B/AI0 (DIFF)", "B/AI1 (DIFF)", "B/AI2 (DIFF)", "B/AI3 (DIFF)"] ("AI Channel")
        w72 = T14 [enum."A/AI0"] items=["Not Connected", "AudioIn/Left", "AudioIn/Right", "C/AI0", "C/AI1", "A/AI0", "A/AI1", "A/AI2", "A/AI3", "A/AI4", "A/AI5", "A/AI6", "A/AI7", "B/AI0", "B/AI1", "B/AI2", "B/AI3", "B/AI4", "B/AI5", "B/AI6", "B/AI7", "AI/AI0", "AI/AI1", "AI/AI2", "AI/AI3", "A/AI0 (DIFF)", "A/AI1 (DIFF)", "A/AI2 (DIFF)", "A/AI3 (DIFF)", "B/AI0 (DIFF)", "B/AI1 (DIFF)", "B/AI2 (DIFF)", "B/AI3 (DIFF)"] ("AI Channel")
        # "IR + Ultrasonic Sensor Loop"
        n162 = call <vilib>:"Ping.vi"("Mxp Side"=Mxp_Selection."MXP B") -> ("CM"=w59:fxp<+,64,16>)  [unwired: 8 in, 2 out]
        "CM" <- w59
        n163 = call <vilib>:"Sharp IR.vi"("AI Channel"=w72) -> ("Sharp IR Distance"=→"Right IR Sensor":dbl)  [unwired: 8 in, 2 out]
        n164 = call <vilib>:"Sharp IR.vi"("AI Channel"=w71) -> ("Sharp IR Distance"=→"Left IR Sensor":dbl)  [unwired: 8 in, 2 out]
        n165 = Greater Or Equal?(x=w59, y=fxp<+,64,16> 299.0) -> (x >= y?=w62:bool)
        n166 = call <vilib>:"Mean PtByPt.vi"("x"=w59, "sample length"=100) -> ()  [unwired: 2 in, 2 out]
        n167 = Select(t=w61, s=w62, f=w59) -> (s? t:f=w60:fxp<+,64,16>)
        "Ultrasonic sensor" <- w60
        n168 = call "FGV Stop.vi"("Init/Read/Write State"=States_for_Action_Engine."Read") -> ("Output node"=w66:bool)  [unwired: 2 in, 1 out]
        n169 = In Range and Coerce(upper limit=fxp<+,64,16> 250.0, x=w59, lower limit=fxp<+,64,16> 0.0 ("CM")) -> ()  [unwired: 2 out]
        n170 = Wait Until Next ms Multiple(millisecond multiple=u32 10) -> ()  [unwired: 1 out]
      }
      n171 = call <vilib>:"NavX Close.vi"("NavX Info In"=w3) -> ()  [unwired: 10 in, 1 out]
      n172 = call <vilib>:"NavX Close.vi"("NavX Info In"=w7) -> ()  [unwired: 10 in, 1 out]
      n173 = call <vilib>:"NavX Close.vi"("NavX Info In"=w6) -> ()  [unwired: 10 in, 1 out]
      n174 = call <vilib>:"NavX Close.vi"("NavX Info In"=w5) -> ()  [unwired: 10 in, 1 out]
      n175 = call <vilib>:"NavX Close.vi"("NavX Info In"=w4) -> ()  [unwired: 10 in, 1 out]
      n176 = Merge Errors "Merge Errors"(w31, w30) -> (w10:errorcluster)
      n177 = Merge Errors(w16, w10) -> (w12:errorcluster)
      n178 = Destroy User Event(user event=w34, error in=w12) -> ()  [unwired: 1 out]
      n179 = Destroy User Event(user event=w35, error in=w12) -> ()  [unwired: 1 out]
      n180 = Unregister For Events(event registration refnum=w26, error in=w12) -> ()  [unwired: 1 out]
      n181 = Release Queue(queue=w25, error in (no error)=w12) -> ()  [unwired: 1 in, 3 out]
      n182 = Release Queue(queue=w11, error in (no error)=w12) -> ()  [unwired: 1 in, 3 out]
    }
  }
